vi "Options.vi"(11 "DataCluster in":T1={"Core"={"Current VI Reference"=refnum, "Close Panel on Exit?"=FALSE, "Exit"=FALSE}, "Connections"={"Arduino"={"VISA"="", "Data Feed"="", "Connected"=FALSE}, "Ready"=FALSE}, "Files"={"Path"=path "", "Filename"="", "File List"=1, "Buffer"={"Buffer"=refnum, "Size"=1}, "Downloading"=FALSE}}) -> (3 "DataCluster out":T1={"Core"={"Current VI Reference"=refnum, "Close Panel on Exit?"=FALSE, "Exit"=FALSE}, "Connections"={"Arduino"={"VISA"="", "Data Feed"="", "Connected"=FALSE}, "Ready"=FALSE}, "Files"={"Path"=path "", "Filename"="", "File List"=1, "Buffer"={"Buffer"=refnum, "Size"=1}, "Downloading"=FALSE}})   [LabVIEW 2022 SP3]
uses:
  DataCluster.ctl
panel:
  in  "Timing Mode":i32(ring)=14713 items=["Automatic"=16097, "High Resolution"=10195, "High Speed"=14712, "Best 50 Hz Rejection"=14713, "Best 60 Hz Rejection"=14714, "Custom"=10137]
  in  "Derivative time":dbl min=0.0 format="%.3f min"
  in  "Integral time":dbl=0.01 min=0.0 format="%.3f min"
  in  "Proportional gain":dbl=1.0 min=0.0 format="%.3f"
  in  "Control Sample Rate":i32=1 min=1 max=20 step=1 format="%.0f Samples/sec"
  in  "Cancel":bool
  in  "OK":bool
  in  "Sample Size":i32=1 min=1 max=200 step=1
  in  "Buffer Size":i32=1 min=1 max=300 step=1
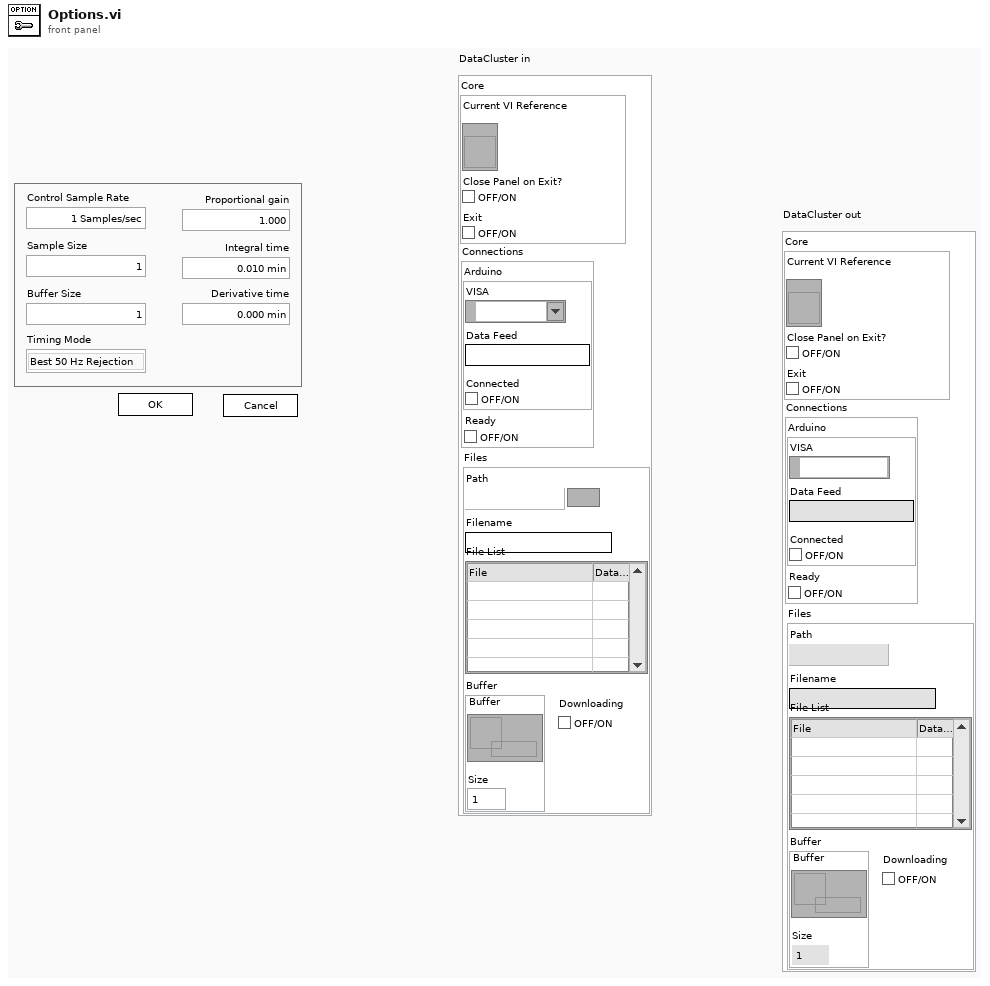
[diagram p1: front panel]
types:
  T1 = typedef "DataCluster.ctl" = cluster{"Core":cluster{"Current VI Reference":refnum<vi>, "Close Panel on Exit?":bool, "Exit":bool}, "Connections":cluster{"Arduino":cluster{"VISA":refnum<visa-resource-name>, "Data Feed":string, "Connected":bool}, "Ready":bool}, "Files":cluster{"Path":path, "Filename":string, "File List":i32, "Buffer":cluster{"Buffer":refnum<queue>, "Size":i32}, "Downloading":bool}}
  T2 = enum8{"Enabled", "Disabled", "Disabled and Grayed Out"}
  T3 = cluster{"proportional gain (Kc)":dbl, "integral time (Ti, min)":dbl, "derivative time (Td, min)":dbl}
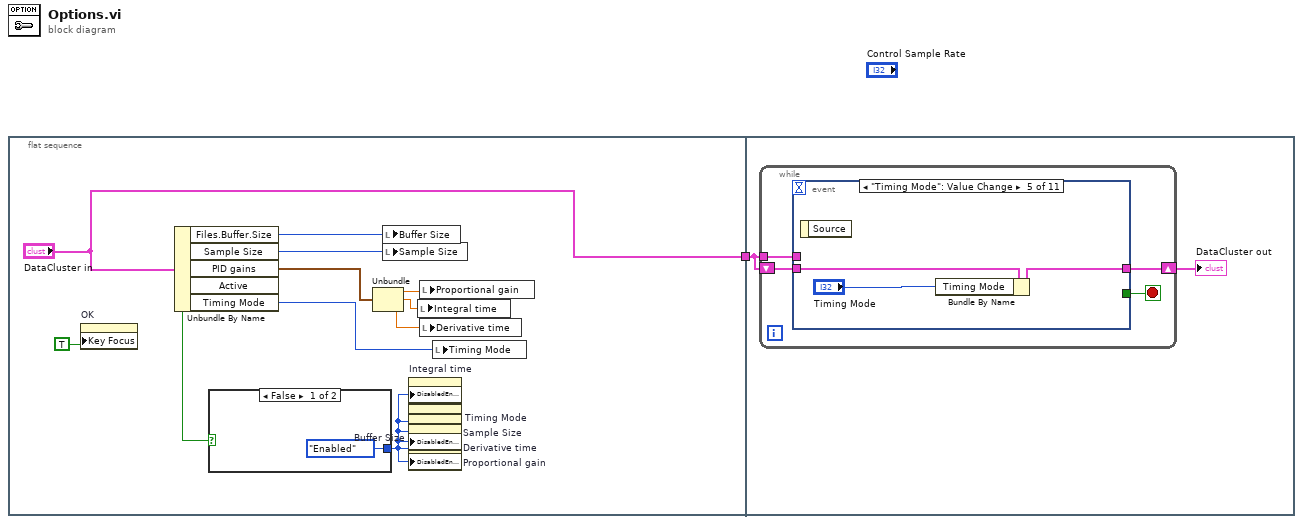
[diagram p0: block diagram]
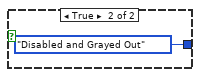
[diagram p2: hidden frame]
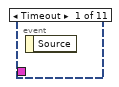
[diagram p3: hidden frame]
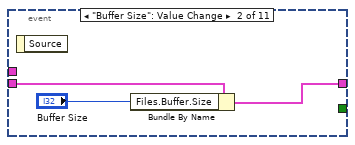
[diagram p4: hidden frame]
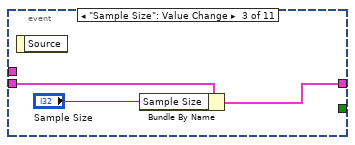
[diagram p5: hidden frame]
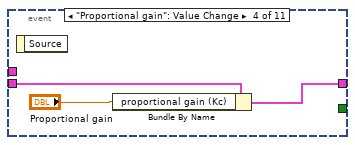
[diagram p6: hidden frame]
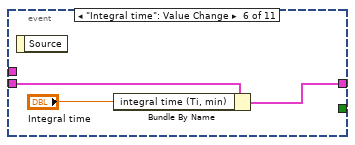
[diagram p7: hidden frame]
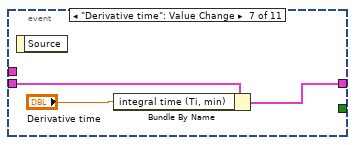
[diagram p8: hidden frame]
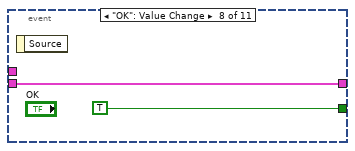
[diagram p9: hidden frame]
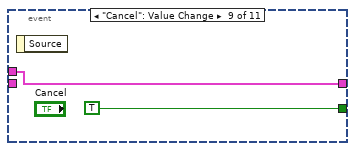
[diagram p10: hidden frame]
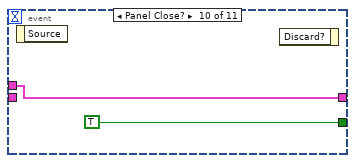
[diagram p11: hidden frame]
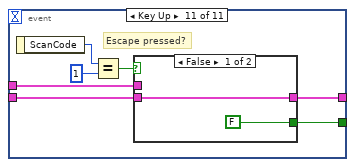
[diagram p12: hidden frame]
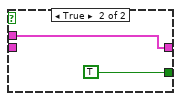
[diagram p13: hidden frame]
diagram:
  n1 = flat-sequence {
    tunnel: ["DataCluster in"] -> w1
    tunnel: w1 -> [w16]
    frame #0 {
      n2 = property on="OK" class="Bool"("Key Focus"=TRUE) -> ()  [unwired: 2 in, 2 out]
      n3 = Unbundle By Name("DataCluster in") -> ("Files.Buffer.Size"=w10:i32, "Sample Size"=w9:i32, "PID gains"=w7:T3, "Active"=w8:bool, "Timing Mode"=w2:i32)
      n4 = case shown="False" w8 {
        tunnel: [T2."Enabled" ("Disabled") T2."Disabled and Grayed Out" ("Disabled")] -> w3
        frame False {
        }
        frame True {
        }
      }
      n5 = Unbundle(w7) -> ("proportional gain (Kc)"=w6:dbl, "integral time (Ti, min)"=w5:dbl, "derivative time (Td, min)"=w4:dbl)
      n6 = local write "Buffer Size"(w10) -> ()
      n7 = local write "Sample Size"(w9) -> ()
      n8 = property on="Integral time" class="DigNum (strict)"("DisabledEnum"=w3) -> ()  [unwired: 2 in, 2 out]
      n9 = property on="Timing Mode" class="Ring (strict)"("DisabledEnum"=w3) -> ()  [unwired: 2 in, 2 out]
      n10 = property on="Sample Size" class="DigNum (strict)"("DisabledEnum"=w3) -> ()  [unwired: 2 in, 2 out]
      n11 = property on="Buffer Size" class="DigNum (strict)"("DisabledEnum"=w3) -> ()  [unwired: 2 in, 2 out]
      n12 = property on="Derivative time" class="DigNum (strict)"("DisabledEnum"=w3) -> ()  [unwired: 2 in, 2 out]
      n13 = property on="Proportional gain" class="DigNum (strict)"("DisabledEnum"=w3) -> ()  [unwired: 2 in, 2 out]
      n14 = local write "Integral time"(w5) -> ()
      n15 = local write "Proportional gain"(w6) -> ()
      n16 = local write "Derivative time"(w4) -> ()
      n17 = local write "Timing Mode"(w2) -> ()
    }
    frame #1 {
      n18 = while {
        shift-right: [w20] -> w15
        shift-left: w16 -> [w19]
        tunnel: w16 -> [w18]
        stop <- w17 stop-if-true
        n19 = event shown="[4] \"Timing Mode\": Value Change" {
          selector: _ -> [_ _ _ _ _ _ _ _ _ _ _]
          dyn-events: _ -> [_ _ _ _ _ _ _ _ _ _ _]
          timeout: _ -> [_ _ _ _ _ _ _ _ _ _ _]
          tunnel: w19 -> [_ w23 w26 w29 w32 w35 w38 w40 _ _ w45]
          tunnel: [_ w22 w25 w28 w31 w34 w37 w40 w42 w44 w47] -> w20
          tunnel: w18 -> [_ _ _ _ _ _ _ _ w42 w44 w46]
          tunnel: [_ _ _ _ _ _ _ TRUE TRUE TRUE w51] -> w17
          event Timeout {
            n20 = event-data() -> ()  [unwired: 1 in, 1 out]
          }
          event "Buffer Size": Value Change {
            n21 = event-data() -> ()  [unwired: 1 in, 1 out]
            n22 = Bundle By Name(cluster=w23, "Files.Buffer.Size"="Buffer Size") -> (w22:T1)
          }
          event "Sample Size": Value Change {
            n23 = event-data() -> ()  [unwired: 1 in, 1 out]
            n24 = Bundle By Name(cluster=w26, "Sample Size"="Sample Size") -> (w25:T1)
          }
          event "Proportional gain": Value Change {
            n25 = event-data() -> ()  [unwired: 1 in, 1 out]
            n26 = Bundle By Name(cluster=w29, "proportional gain (Kc)"="Proportional gain") -> (w28:T1)
          }
          event "Timing Mode": Value Change {
            n27 = event-data() -> ()  [unwired: 1 in, 1 out]
            n28 = Bundle By Name(cluster=w32, "Timing Mode"="Timing Mode") -> (w31:T1)
          }
          event "Integral time": Value Change {
            n29 = event-data() -> ()  [unwired: 1 in, 1 out]
            n30 = Bundle By Name(cluster=w35, "integral time (Ti, min)"="Integral time") -> (w34:T1)
          }
          event "Derivative time": Value Change {
            n31 = event-data() -> ()  [unwired: 1 in, 1 out]
            n32 = Bundle By Name(cluster=w38, "integral time (Ti, min)"="Derivative time") -> (w37:T1)
          }
          event "OK": Value Change {
            n33 = event-data() -> ()  [unwired: 1 in, 1 out]
          }
          event "Cancel": Value Change {
            n34 = event-data() -> ()  [unwired: 1 in, 1 out]
          }
          event Panel Close? {
            n35 = event-data() -> ()  [unwired: 1 in, 1 out]
            n36 = event-data() -> ()  [unwired: 2 in, 1 out]
          }
          event Key Up {
            # "Escape pressed?"
            n37 = event-data() -> ("ScanCode"=w50:i16)  [unwired: 1 in]
            n38 = Equal?(x=w50, y=i16 1) -> (x = y?=w48:bool)
            n39 = case shown="False" w48 {
              tunnel: [FALSE TRUE] -> w51
              tunnel: [w53 w54] -> w47
              tunnel: w46 -> [_ w54]
              tunnel: w45 -> [w53 _]
              frame False {
              }
              frame True {
              }
            }
          }
        }
      }
      "DataCluster out" <- w15
    }
  }
